vi "Read ipAddress.vi"(8 "error in (no error)":errorcluster, 11 "MelsecTCP in":refnum<class "MelsecMcNet.lvclass">) -> (0 "error out":errorcluster, 2 "ipAddress":string, 3 "MelsecTCP out":refnum<class "MelsecMcNet.lvclass">)   [LabVIEW 2020, in "MelsecMcNet.lvclass"]
uses:
  MelsecMcNet.lvclass
  MelsecMcNet.lvclass/MelsecMcNet.ctl
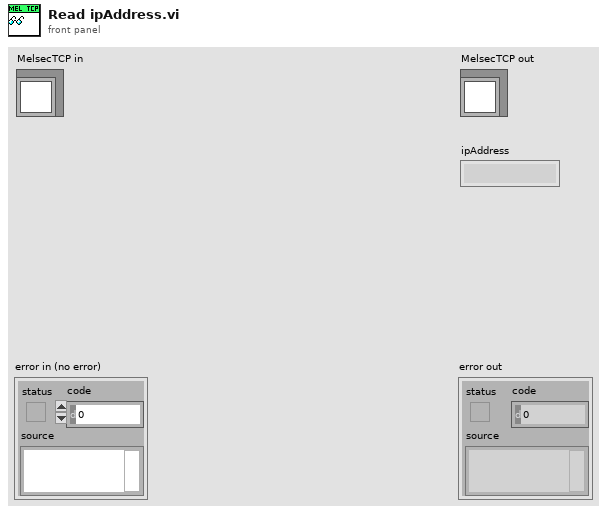
[diagram p1: front panel]
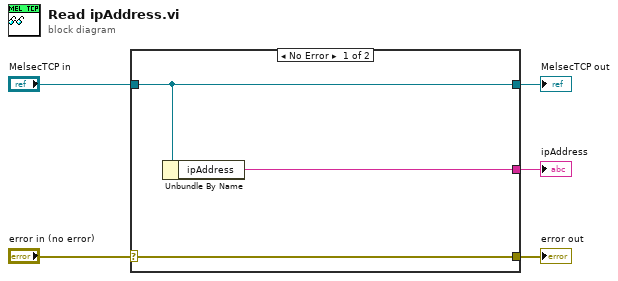
[diagram p0: block diagram]
diagram:
  n1 = case shown="No Error" "error in (no error)" {
    selector: "error in (no error)" -> [w8 w9]
    tunnel: [w8 w9] -> w4
    tunnel: [w7 w10] -> w2
    tunnel: "MelsecTCP in" -> [w7 w10]
    tunnel: [w6 _] -> w1
    frame No Error {
      n2 = Unbundle By Name(w7) -> ("ipAddress"=w6:string)
    }
    frame Error {
    }
  }
  "error out" <- w4
  "MelsecTCP out" <- w2
  "ipAddress" <- w1
